vi "ReceiveMultipleStrings.vi"(8 "error in (no error)":errorcluster, 9 "waiting time ms (-1: forever)":i32, 10 "keep semaphore":bool, 11 "queue cluster":T1) -> (0 "error out":errorcluster, 1 "new value":bool, 2 "received strings":string[](array[string]), 3 "queue cluster out":T1)   [LabVIEW 2014]
uses:
  typedefs/QueueCluster.ctl
  typedefs/clientStatus.ctl
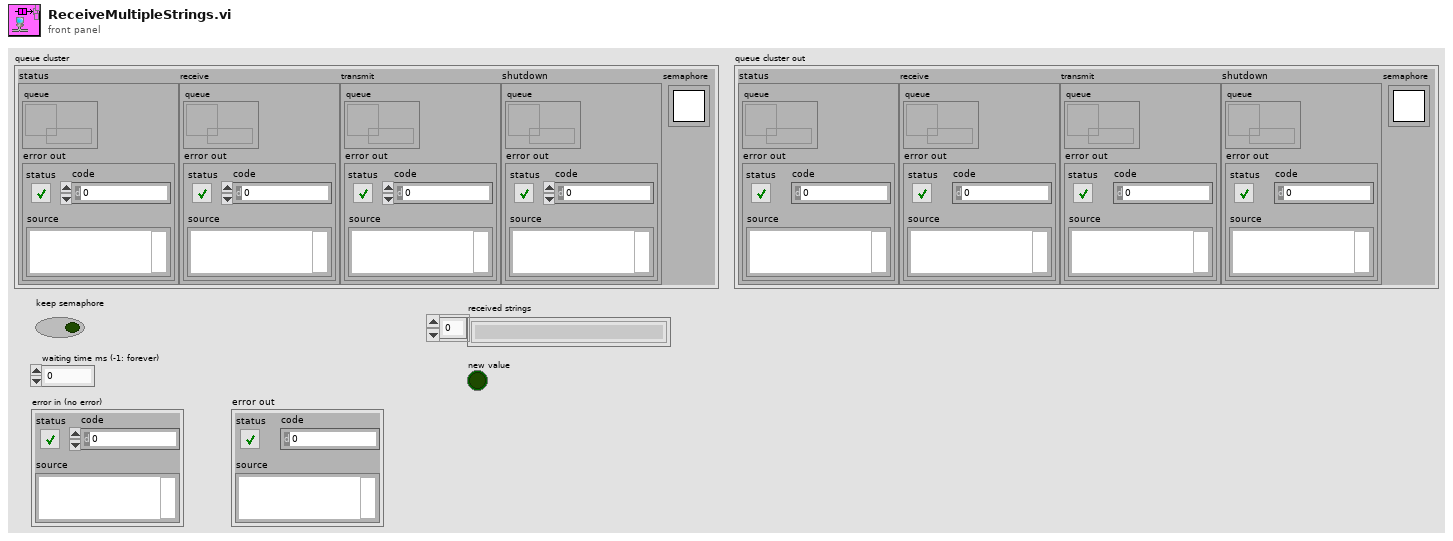
[diagram p1: front panel]
types:
  T1 = typedef "QueueCluster.ctl" = cluster{"status":cluster{"queue":refnum<queue>, "error out":errorcluster}, "receive":cluster{"queue":refnum<queue>, "error out":errorcluster}, "transmit":cluster{"queue":refnum<queue>, "error out":errorcluster}, "shutdown":cluster{"queue":refnum<queue>, "error out":errorcluster}, "semaphore":T2}
  T2 = typedef "Semaphore RefNum" = refnum<k1>
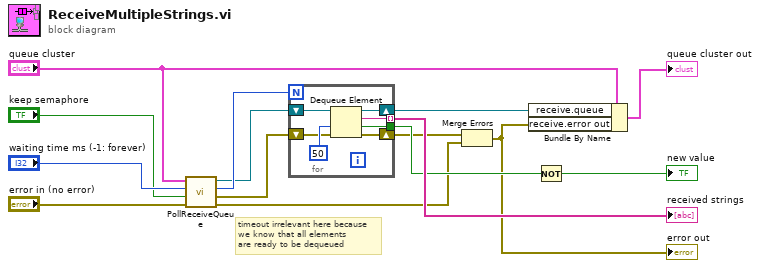
[diagram p0: block diagram]
diagram:
  # "timeout irrelevant here because\nwe know that all elements \nare ready to be dequeued"
  n1 = call "PollReceiveQueue.vi"("error in (no error)"="error in (no error)", "keep semaphore"="keep semaphore", "waiting time ms (-1: forever)"="waiting time ms (-1: forever)", "queue cluster"="queue cluster") -> ("semaphore error out"=w3:errorcluster, "receive queue error out"=w2:errorcluster, "# elements in queue"=w7:i32, "receive queue"=w1:refnum<queue>)  [unwired: 4 in]
  n2 = for {
    N: w7 -> [_]
    tunnel: [w20] -> w11 mode=indexing
    tunnel: [w17] -> w8
    shift-right: [w22] -> w13
    shift-left: w1 -> [w21]
    shift-right: [w19] -> w5
    shift-left: w2 -> [w16]
    n3 = Dequeue Element(queue=w21, timeout in ms (-1)=50, error in (no error)=w16) -> (queue out=w22:refnum<queue>, element=w20:string, timed out?=w17:bool, error out=w19:errorcluster)
  }
  "received strings" <- w11
  n4 = Merge Errors(w5, w3) -> (w4:errorcluster)
  "error out" <- w4
  n5 = Bundle By Name(cluster="queue cluster", "receive.queue"=w13, "receive.error out"=w4) -> (→"queue cluster out":T1)
  n6 = Not(x=w8) -> (.not. x?=→"new value":bool)
